vi "OnDemand_VoltageOutput.vi"(6 "Channel Array":dbl[](array[slide]) scale=0.0..5.067, 8 "SampClk.Rate 2":dbl, 9 "minimum voltage":dbl=-5.0 format="%0.2f", 10 "maximum voltage":dbl=5.0 format="%0.2f", 11 "physical channels":tag) -> (0 "error out":errorcluster, 1 "SampClk.Rate":dbl, 2 "number of samples written per channel":u32)   [LabVIEW 2022 SP3]
uses:
  <vilib>/DAQmx/write.llb/DAQmx Write (Analog 1D DBL NChan 1Samp).vi
  <vilib>/DAQmx/create/channels.llb/DAQmx Create Channel (AO-Voltage-Basic).vi
  <vilib>/DAQmx/miscellaneous.llb/DAQmx Fill In Error Info.vi
  <resource>/objmgr/daqmx.rc
panel:
  # "VOLTAGE OUTPUT"
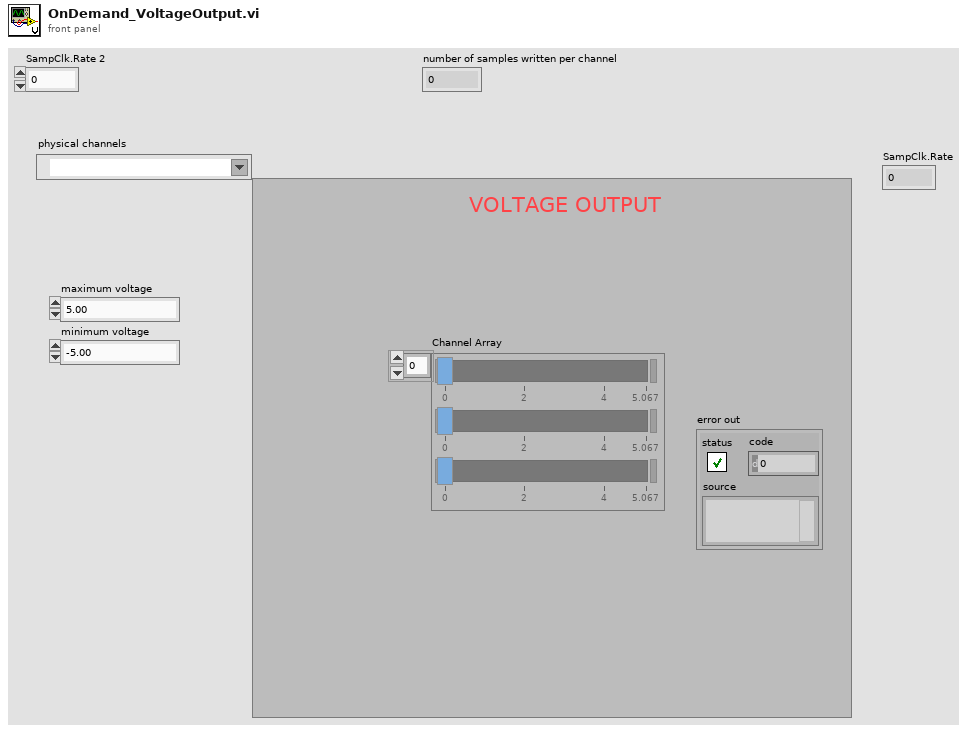
[diagram p1: front panel]
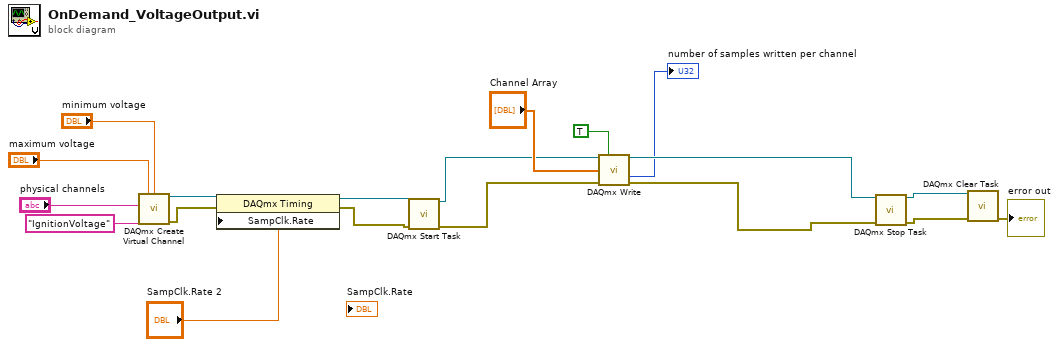
[diagram p0: block diagram]
diagram:
  n1 = call-poly <vilib>:"DAQmx Create Virtual Channel.vi"("maximum value"="maximum voltage", "minimum value"="minimum voltage", "physical channels"="physical channels", "name to assign"="IgnitionVoltage") -> ("task out"=w5:refnum<k21>, "error out"=w4:errorcluster)  [unwired: 10 in]
  n2 = property class="DAQmx Timing"(reference=w5, error in=w4, "SampClk.Rate"="SampClk.Rate 2") -> (reference out=w6:refnum<k21>, error out=w7:errorcluster)
  n3 = call <vilib>:"DAQmx Start Task.vi"("task/channels in"=w6, "error in"=w7) -> ("task out"=w13:refnum<k21>, "error out"=w12:errorcluster)  [unwired: 12 in]
  n4 = call-poly <vilib>:"DAQmx Write.vi"("task/channels in"=w13, "auto start"=TRUE, "data"="Channel Array", "error in"=w12) -> ("task out"=w11:refnum<k21>, "number of samples written per channel"=→"number of samples written per channel":u32, "error out"=w10:errorcluster)  [unwired: 9 in]
  n5 = call <vilib>:"DAQmx Stop Task.vi"("task/channels in"=w11, "error in"=w10) -> ("task out"=w17:refnum<k21>, "error out"=w16:errorcluster)  [unwired: 12 in]
  n6 = call <vilib>:"DAQmx Clear Task.vi"("task in"=w17, "error in"=w16) -> ("error out"=→"error out":errorcluster)  [unwired: 13 in]
